vi "Set Scan Rate.vi"(0 "Notifier Name":string, 7 "Scan Rate (Hz)":dbl, 11 "Error In":errorcluster) -> (4 "Notifier Name Dup":string, 8 "Success":bool, 15 "Error Out":errorcluster)   [LabVIEW 2020]
uses:
  3 Mirror Scan Type Defs/3 Mirror Scan Note Type.ctl
  3 Mirror Scan Type Defs/3 Mirror Scan Actions.ctl
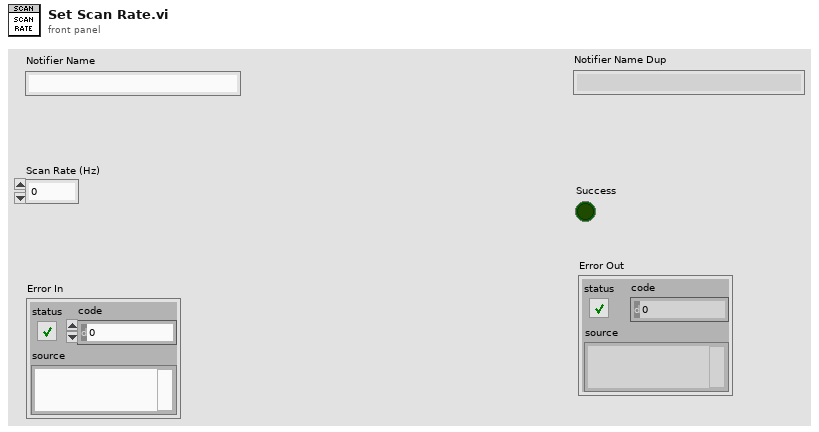
[diagram p1: front panel]
types:
  T1 = typedef "3 Mirror Scan Note Type.ctl" = cluster{"Actions":T2, "Global Rectangle":i32[], "Running":bool, "Scan Frequency (Hz)":dbl, "Scan Time (s)":dbl}
  T2 = typedef "3 Mirror Scan Actions.ctl" = enum16{"Idle", "Scan Timed", "Scan Live", "Convert ROI", "Run Scan", "Exit Loop", "Quit"}
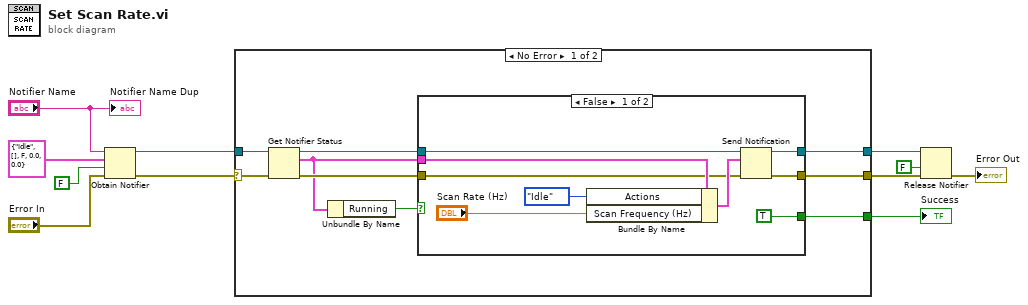
[diagram p0: block diagram]
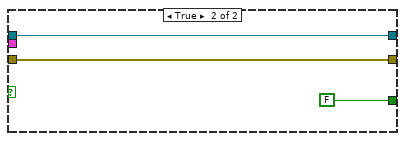
[diagram p2: hidden frame]
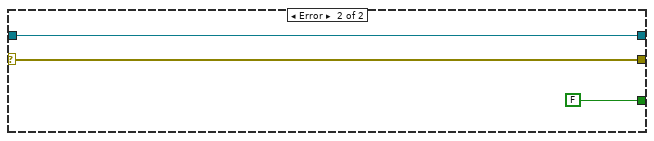
[diagram p3: hidden frame]
diagram:
  n1 = Obtain Notifier(name (unnamed)="Notifier Name", notification data type=T1 {"Actions"=enum."Idle", "Global Rectangle"=[], "Running"=FALSE, "Scan Frequency (Hz)"=0.0, "Scan Time (s)"=0.0} ("3 Mirror Notifier"), create if not found? (T)=FALSE, error in (no error)="Error In") -> (notifier out=w7:refnum<notifier>, error out=w8:errorcluster)  [unwired: 1 out]
  n2 = case shown="No Error" w8 {
    selector: w8 -> [w19 w34]
    tunnel: w7 -> [w20 w35]
    tunnel: [w14 w35] -> w5
    tunnel: [w13 w34] -> w3
    tunnel: [w12 FALSE] -> w1
    frame No Error {
      n3 = Get Notifier Status(notifier=w20, error in (no error)=w19) -> (notifier out=w16:refnum<notifier>, current notification=w15:T1, error out=w17:errorcluster)  [unwired: 2 out]
      n4 = Unbundle By Name(w15) -> ("Running"=w18:bool)
      n5 = case shown="False" w18 {
        tunnel: w17 -> [w24 w31]
        tunnel: w16 -> [w26 w32]
        tunnel: w15 -> [w29 _]
        tunnel: [w23 w32] -> w14
        tunnel: [w22 w31] -> w13
        tunnel: [TRUE FALSE] -> w12
        frame False {
          n6 = Bundle By Name(cluster=w29, "Actions"=3_Mirror_Scan_Actions."Idle", "Scan Frequency (Hz)"="Scan Rate (Hz)") -> (w25:T1)
          n7 = Send Notification(notification=w25, notifier=w26, error in (no error)=w24) -> (notifier out=w23:refnum<notifier>, error out=w22:errorcluster)
        }
        frame True {
        }
      }
    }
    frame Error {
    }
  }
  "Success" <- w1
  n8 = Release Notifier(notifier=w5, force destroy? (F)=FALSE, error in (no error)=w3) -> (error out=→"Error Out":errorcluster)  [unwired: 2 out]
  "Notifier Name Dup" <- "Notifier Name"
